vi "Pattern Generator (Block Approach).vi"(7 "sampling info":cluster{"Fs":dbl, "#s":dbl}={"Fs"=250000000.0, "#s"=1000.0} {"Fs" format="%#_p"}, 9 "Loop Rate (kHz)":dbl=100.0, 10 "Marker Position":u16, 11 "Frequency":dbl=10.0 format="%0.2p") -> (2 "Trigger":bool, 3 "Data":i16(graph))   [LabVIEW 2011]
uses:
  <vilib>/measure/NI_MABase.lvlib
panel:
  in  "stop":bool
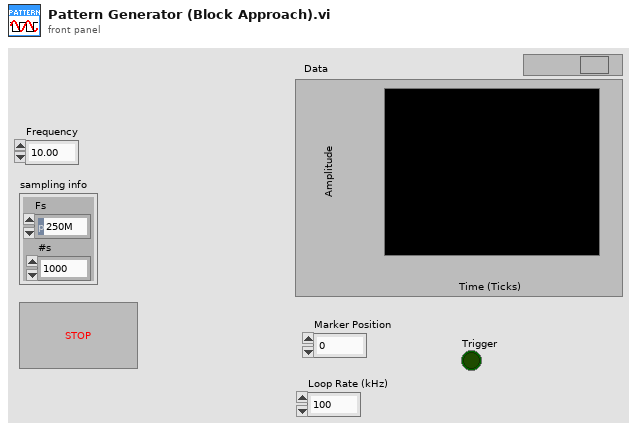
[diagram p1: front panel]
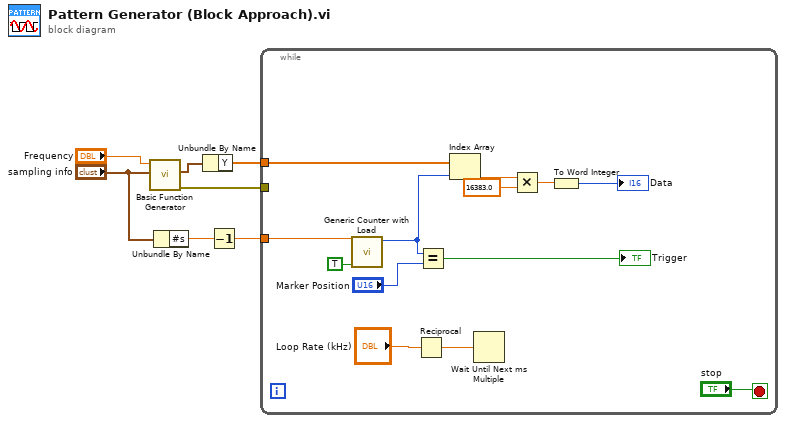
[diagram p0: block diagram]
diagram:
  n1 = call <vilib>:"Basic Function Generator.vi"("sampling info"="sampling info", "frequency"="Frequency") -> ("error out"=w5:errorcluster, "signal out"=w4:waveform(dbl))  [unwired: 7 in, 1 out]
  n2 = Unbundle By Name("sampling info") -> ("#s"=w2:dbl)
  n3 = Unbundle By Name(w4) -> ("Y"=w3:dbl[])
  n4 = Decrement(x=w2) -> (x-1=w1:dbl)
  n5 = while {
    tunnel: w5 -> [_]
    tunnel: w3 -> [w19]
    tunnel: w1 -> [w18]
    stop <- "stop" stop-if-true
    n6 = call "Generic Counter with Load.vi"("INC?"=TRUE, "rollover"=w18) -> ("count"=w11:u16)  [unwired: 9 in]
    n7 = Reciprocal(x="Loop Rate (kHz)") -> (1/x=w8:dbl)
    n8 = Equal?(x=w11, y="Marker Position") -> (x = y?=→"Trigger":bool)
    n9 = Index Array(array=w19, index=w11) -> (element=w15:dbl)
    n10 = Wait Until Next ms Multiple(millisecond multiple=w8) -> ()  [unwired: 1 out]
    n11 = Multiply(x=w15, y=16383.0) -> (x*y=w13:dbl)
    n12 = To Word Integer(number=w13) -> (16bit integer=→"Data":i16)
  }
